vi "ASI_move_mosaic.vi"(1 "Mosaic cluster":cluster{dbl[], dbl[]}[](array[cluster]), 2 "VISA resource name":refnum<visa-resource-name>="COM7", 3 "error in":errorcluster, 4 "XY mosaic":dbl[](array[numeric]), 5 "XY positions timelapse":refnum<vi>) -> (0 "error out":errorcluster)   [LabVIEW 2015]
uses:
  <vilib>/Instr/_visa.llb/VISA Flush IO Buffer Mask.ctl
  GLOBAL/Global_CAMERA_TYPE.vi
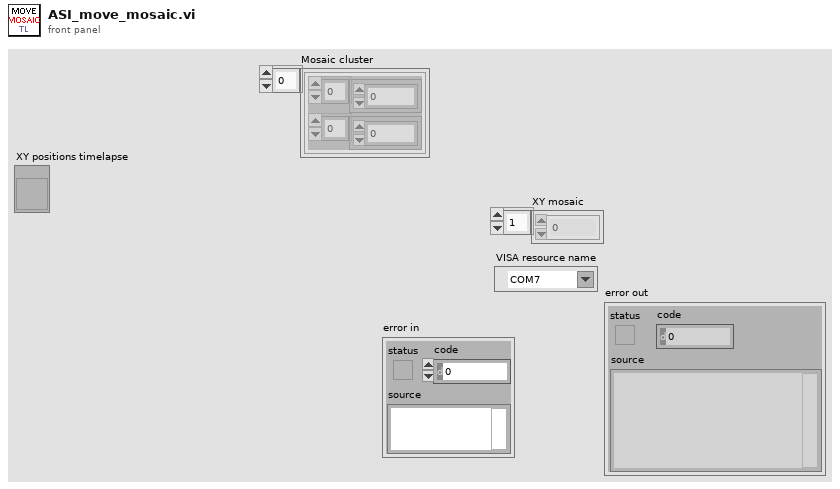
[diagram p1: front panel]
types:
  T1 = typedef "VISA Flush IO Buffer Mask.ctl" = u16
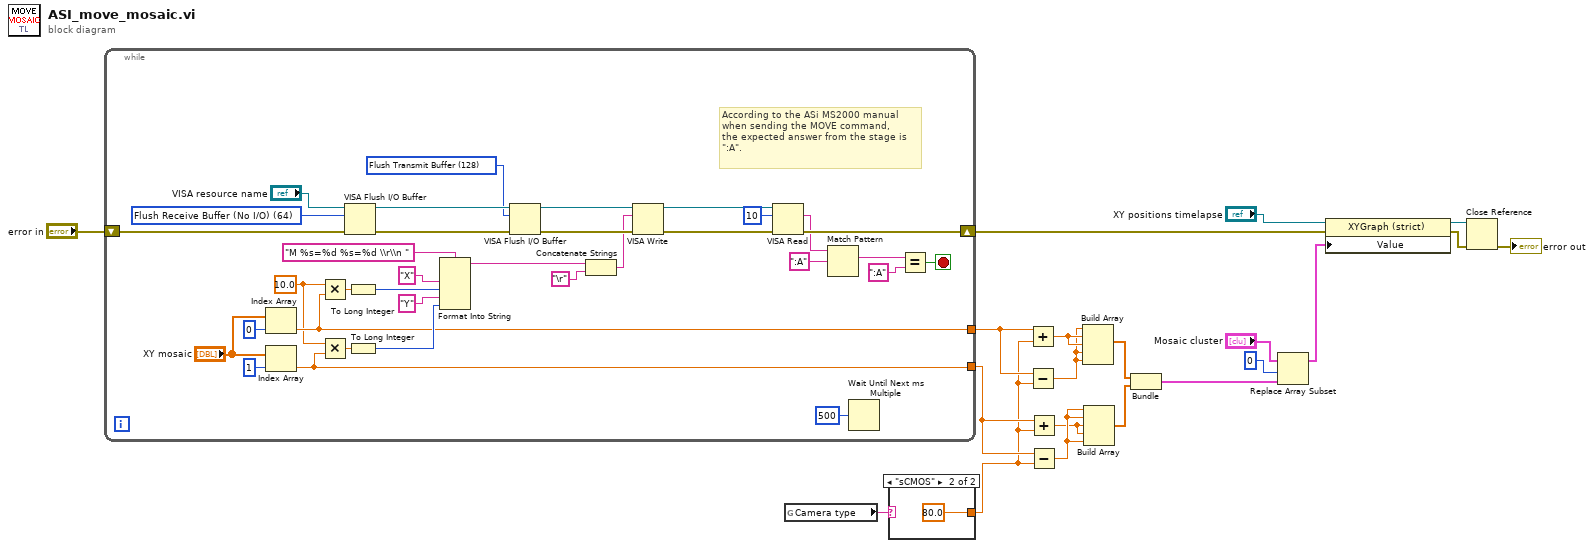
[diagram p0: block diagram]
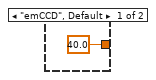
[diagram p2: hidden frame]
diagram:
  n1 = while {
    shift-right: [w34] -> w11
    shift-left: "error in" -> [w42]
    tunnel: [w24] -> w17
    tunnel: [w22] -> w16
    stop <- w29 stop-if-true
    w23 = 10.0 ("x")
    w45 = T1 128 items=["Flush Receive Buffer"=16, "Write Transmit Buffer to Device"=32, "Flush Receive Buffer (No I/O)"=64, "Flush Transmit Buffer"=128] ("Mask")
    w48 = T1 64 items=["Flush Receive Buffer"=16, "Write Transmit Buffer to Device"=32, "Flush Receive Buffer (No I/O)"=64, "Flush Transmit Buffer"=128] ("Mask")
    # "According to the ASi MS2000 manual\nwhen sending the MOVE command, \nthe expected answer from the stage is\n\":A\"."
    n2 = Index Array(array="XY mosaic", index=0 ("index (row)")) -> (element=w24:dbl)
    n3 = Index Array(array="XY mosaic", index=1 ("index (row)")) -> (element=w22:dbl)
    n4 = Multiply(x=w23, y=w24) -> (x*y=w25:dbl)
    n5 = Multiply(x=w23, y=w22) -> (x*y=w21:dbl)
    n6 = VISA Flush I/O Buffer(VISA resource name="VISA resource name", mask (16)=w48, error in (no error)=w42) -> (VISA resource name out=w46:refnum<visa-resource-name>, error out=w47:errorcluster)
    n7 = To Long Integer(number=w25) -> (32bit integer=w27:i32)
    n8 = To Long Integer(number=w21) -> (32bit integer=w26:i32)
    n9 = Format Into String "Format Into String"(format string="M %s=%d %s=%d \\r\\n ", "X" ("Axis"), w27, "Y" ("Axis"), w26) -> (resulting string=w40:string)  [unwired: 2 in, 1 out]
    n10 = VISA Flush I/O Buffer(VISA resource name=w46, mask (16)=w45, error in (no error)=w47) -> (VISA resource name out=w43:refnum<visa-resource-name>, error out=w44:errorcluster)
    n11 = Concatenate Strings(w40, "\r") -> (w38:string)
    n12 = VISA Write(VISA resource name=w43, write buffer=w38, error in (no error)=w44) -> (VISA resource name out=w51:refnum<visa-resource-name>, error out=w41:errorcluster)  [unwired: 1 out]
    n13 = VISA Read(VISA resource name=w51, byte count=u32 10, error in (no error)=w41) -> (read buffer=w28:string, error out=w34:errorcluster)  [unwired: 2 out]
    n14 = Match Pattern(string=w28, regular expression=":A" ("y")) -> (match substring=w31:string)  [unwired: 1 in, 3 out]
    n15 = Wait Until Next ms Multiple(millisecond multiple=u32 500) -> ()  [unwired: 1 out]
    n16 = Equal?(x=w31, y=":A") -> (x = y?=w29:bool)
  }
  n17 = global read "Global_CAMERA_TYPE.vi" "Camera type"() -> (w9:string)
  n18 = case shown="\"sCMOS\"" w9 {
    tunnel: [40.0 ("y") 80.0 ("y")] -> w8
    frame "emCCD", Default {
    }
    frame "sCMOS" {
    }
  }
  n19 = Add(x=w17, y=w8) -> (x+y=w13:dbl)
  n20 = Subtract(x=w17, y=w8) -> (x-y=w12:dbl)
  n21 = Add(x=w16, y=w8) -> (x+y=w14:dbl)
  n22 = Subtract(x=w16, y=w8) -> (x-y=w15:dbl)
  n23 = Build Array(w12, w13, w13, w12, w12) -> (w18:dbl[])
  n24 = Build Array(w15, w15, w14, w14, w15) -> (w19:dbl[])
  n25 = Bundle(w18, w19) -> (w6:cluster{dbl[], dbl[]})  [unwired: 1 in]
  n26 = Replace Array Subset(array="Mosaic cluster", new element=w6, index=0) -> (w4:cluster{dbl[], dbl[]}[])
  n27 = property class="XYGraph (strict)"(reference="XY positions timelapse", error in=w11, "Value"=w4) -> (reference out=w2:refnum<vi>, error out=w3:errorcluster)
  n28 = Close Reference(reference=w2, error in (no error)=w3) -> (error out=→"error out":errorcluster)
